vi "Queue.vi"() -> ()   [LabVIEW 2021]
panel:
  out "# elements in queue":i32
  out "Consumer Loop":dbl(graph)
  out "Producer Loop":dbl(graph)
  in  "stop":bool
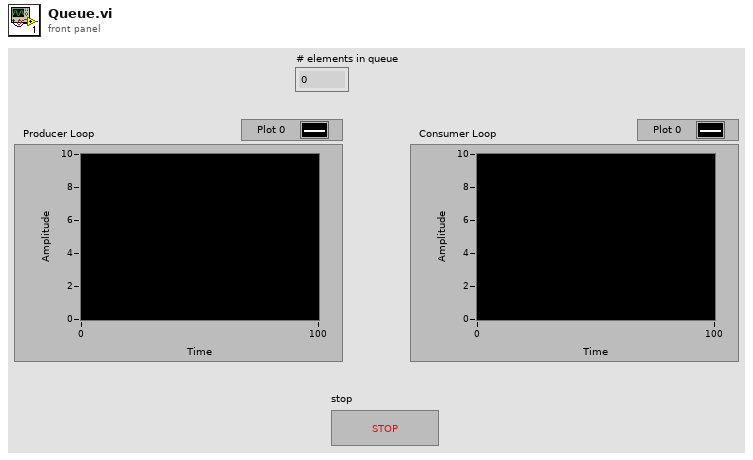
[diagram p1: front panel]
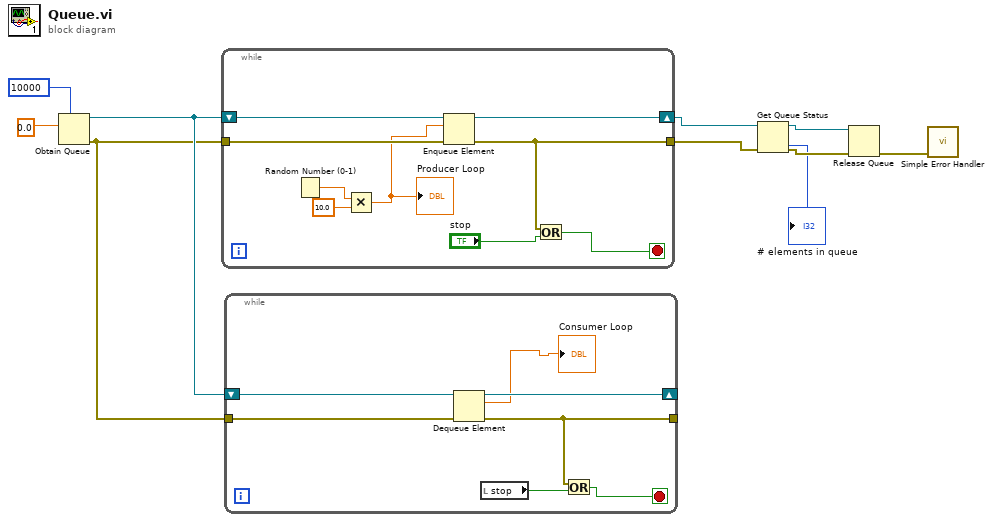
[diagram p0: block diagram]
diagram:
  n1 = Obtain Queue(max queue size (-1, unlimited)=10000, element data type=0.0) -> (queue out=w10:refnum<queue>, error out=w9:errorcluster)  [unwired: 3 in, 1 out]
  n2 = while {
    shift-right: [w18] -> w8
    shift-left: w10 -> [w19]
    tunnel: w9 -> [w17]
    tunnel: [w16] -> w7
    stop <- w15 stop-if-true
    n3 = Random Number (0-1)() -> (number: 0 to 1=w13:dbl)
    n4 = Multiply(x=w13, y=10.0) -> (x*y=w11:dbl)
    "Producer Loop" <- w11
    n5 = Enqueue Element(queue=w19, element=w11, error in (no error)=w17) -> (queue out=w18:refnum<queue>, error out=w16:errorcluster)  [unwired: 1 in, 1 out]
    n6 = Or(x=w16, y="stop") -> (x .or. y?=w15:bool)
  }
  n7 = while {
    shift-right: [w25] -> _
    shift-left: w10 -> [w26]
    tunnel: w9 -> [w24]
    tunnel: [w22] -> _
    stop <- w21 stop-if-true
    n8 = Dequeue Element(queue=w26, error in (no error)=w24) -> (queue out=w25:refnum<queue>, element=→"Consumer Loop":dbl, error out=w22:errorcluster)  [unwired: 1 in, 1 out]
    n9 = local read "stop"() -> (w23:bool)
    n10 = Or(x=w22, y=w23) -> (x .or. y?=w21:bool)
  }
  n11 = Get Queue Status(queue=w8, error in (no error)=w7) -> (queue out=w6:refnum<queue>, error out=w5:errorcluster, # elements in queue=→"# elements in queue":i32)  [unwired: 1 in, 5 out]
  n12 = Release Queue(queue=w6, error in (no error)=w5) -> (error out=w4:errorcluster)  [unwired: 1 in, 2 out]
  n13 = call <vilib>:"Simple Error Handler.vi"("error in (no error)"=w4) -> ()  [unwired: 4 in, 5 out]
